vi "Test Process Unexpected Lifecycle States.vi"(8 "error in (no error)":errorcluster, 11 "Process Test In":refnum<class "Process Dev Test.lvclass">) -> (0 "error out":errorcluster, 3 "Process Test Out":refnum<class "Process Dev Test.lvclass">)   [LabVIEW 2020, in "Process Dev Test.lvclass"]
uses:
  Process Dev Test.lvclass
  C:/Git/astemes-triarc-framework/source/Framework Test/Base Class Test/Base Test.lvclass
  C:/Program Files (x86)/National Instruments/LabVIEW 2020/vi.lib/Astemes/LUnit/Test Case.lvclass
  source/Framework/Process/Process.lvclass
  source/Framework Test Suite/Base Class Test/Base Test.lvclass/Base Test.ctl
  <vilib>/Astemes/LUnit/Test Case.lvclass/Test Case.ctl
  <vilib>/Astemes/LUnit/LUnit Assertion Result.lvclass/LUnit Assertion Result.ctl
  <vilib>/Astemes/LUnit/LUnit Test Case Result.lvclass/LUnit Test Case Result.ctl
  <vilib>/Astemes/LUnit/LUnit Method Result.lvclass/LUnit Method Result.ctl
  source/Framework/Process/Process.lvclass/Process.ctl
  <vilib>/Astemes/LUnit/Palette/Fail.vi
  <vilib>/Astemes/LUnit/Palette/Pass.vi
  <vilib>/Astemes/LUnit/Set Assertion Type.vi
  source/Framework/Process/Private/SubVIs/Wait for finish.vi
  source/Framework/Process/Protected/Messaging/Enqueue Message.vi
  source/Framework/Process/Private/SubVIs/Set Lifecycle State.vi
  source/Framework/Process/Public/Lifecycle/Get Lifecycle State.vi
  <vilib>/Astemes/LUnit/Add test result.vi
  <vilib>/Astemes/LUnit/LUnit Write Passed.vi
  <vilib>/Astemes/LUnit/LUnit Write Message.vi
  <vilib>/Astemes/LUnit/LUnit Write Description.vi
  <vilib>/Astemes/LUnit/LUnit Write Assertion Type.vi
  source/Framework/Process/Private/SubVIs/Handle Debug Data.vi
  <vilib>/Utility/error.llb/Clear Errors.vi
  <vilib>/Astemes/LUnit/LUnit Record Assertion Result.vi
  source/Framework/Logging/Log Debug.vi
  <vilib>/AdvancedString/1D String Array to Delimited String.vi
  <vilib>/Utility/High Resolution Relative Seconds.vi
  <vilib>/Astemes/LUnit/LUnit Aggregate Assertion Results.vi
  <vilib>/Astemes/LUnit/Assertion Result/LUnit Read Status.vi
  <vilib>/Astemes/LUnit/LUnit Read Message.vi
  <vilib>/Astemes/LUnit/LUnit Read Description.vi
  <vilib>/Astemes/LUnit/Method Result/LUnit Merge Status.vi
  <vilib>/Astemes/LUnit/LUnit Concatenate result strings.vi
  <vilib>/Utility/error.llb/Error Cluster From Error Code.vi
  source/Framework/Process/Public/Read Name.vi
  source/Framework/Base/Base.lvclass
  <vilib>/Astemes/LUnit/LUnit Assertion Result.lvclass
  Process Dev Test.lvclass/Process Dev Test.ctl
  <vilib>/Astemes/LUnit/Test Case.lvclass
  source/Framework Test Suite/Base Class Test/Base Test.lvclass
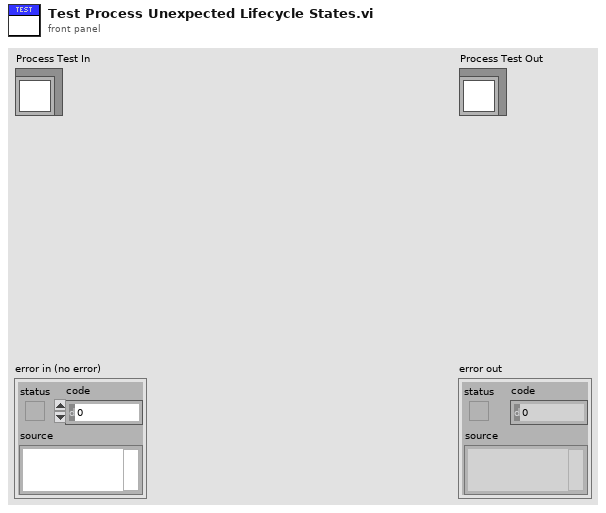
[diagram p1: front panel]
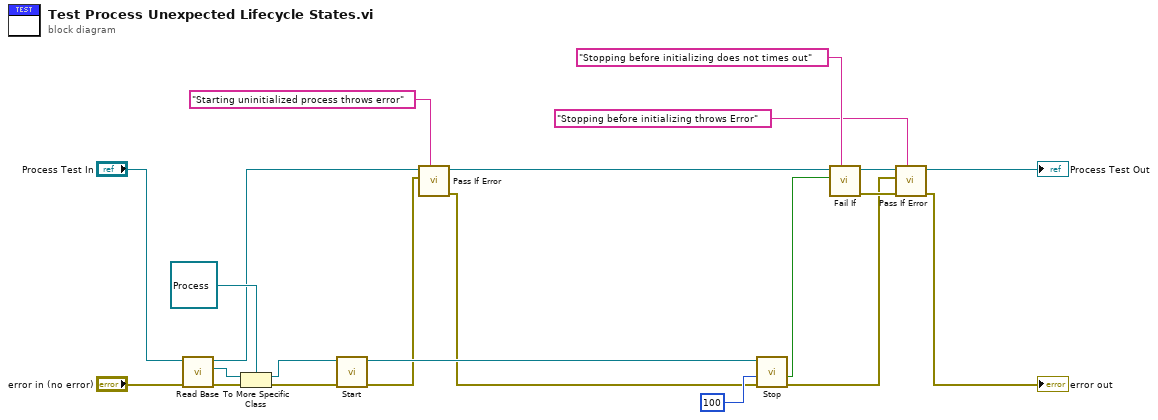
[diagram p0: block diagram]
diagram:
  n1 = call "Read Base.vi"("error in (no error)"="error in (no error)", "Base Class Test In"="Process Test In") -> ("error out"=w8:errorcluster, "Base.lvclass"=w9:refnum<class "Base.lvclass">, "Base Class Test Out"=w4:refnum<class "Process Dev Test.lvclass">)  [unwired: 7 in]
  n2 = To More Specific Class(target class=refnum<class "Process.lvclass"> refnum ("Process.lvclass"), reference=w9, error in=w8) -> (specific class reference=w3:refnum<class "Process.lvclass">, error out=w6:errorcluster)
  n3 = call "Start.vi"("error in (no error)"=w6, "Process In"=w3) -> ("error out"=w18:errorcluster, "Process Out"=w22:refnum<class "Process.lvclass">)  [unwired: 7 in, 1 out]
  n4 = call <vilib>:"Pass If Error.vi"("Description"="Starting uninitialized process throws error", "Assert error"=w18, "LUnit Test Case In"=w4) -> ("error out"=w17:errorcluster, "LUnit Test Case Out"=w20:refnum<class "Process Dev Test.lvclass">)  [unwired: 7 in]
  n5 = call "Stop.vi"("error in (no error)"=w17, "timeout in ms (-1)"=100, "Process In"=w22) -> ("error out"=w2:errorcluster, "timed out?"=w16:bool)  [unwired: 6 in, 1 out]
  n6 = call <vilib>:"Fail If.vi"("Description"="Stopping before initializing does not times out", "Fail?"=w16, "LUnit Test Case In"=w20) -> ("error out"=w13:errorcluster, "LUnit Test Case Out"=w14:refnum<class "Process Dev Test.lvclass">)  [unwired: 7 in]
  n7 = call <vilib>:"Pass If Error.vi"("Description"="Stopping before initializing throws Error", "error in (no error)"=w13, "Assert error"=w2, "LUnit Test Case In"=w14) -> ("error out"=→"error out":errorcluster, "LUnit Test Case Out"=→"Process Test Out":refnum<class "Process Dev Test.lvclass">)  [unwired: 6 in]
